vi "RGB to GRB rev.vi"(9 "ID":u8, 11 "Element":u32) -> (1 "Valid":bool, 2 "Array":bool[](array[boolean]), 3 "Reset":bool)   [LabVIEW 2016]
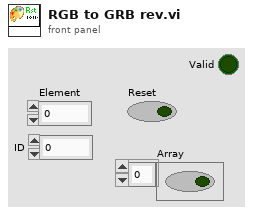
[diagram p1: front panel]
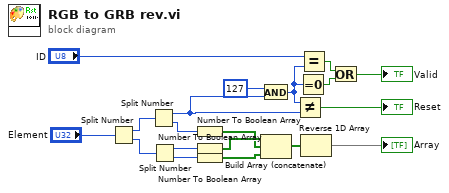
[diagram p0: block diagram]
diagram:
  n1 = Split Number(x="Element") -> (hi(x)=w12:u16, lo(x)=w13:u16)
  n2 = Split Number(x=w12) -> (hi(x)=w9:u8, lo(x)=w14:u8)
  n3 = Split Number(x=w13) -> (hi(x)=w15:u8, lo(x)=w16:u8)
  n4 = Number To Boolean Array(number=w14) -> (Boolean array=w1:bool[])
  n5 = Number To Boolean Array(number=w15) -> (Boolean array=w2:bool[])
  n6 = Number To Boolean Array(number=w16) -> (Boolean array=w17:bool[])
  n7 = And(x=u8 127, y=w9) -> (x .and. y?=w3:u8)
  n8 = Build Array (concatenate)(w2, w1, w17) -> (w18:bool[])
  n9 = Not Equal?(x=w3, y=w9) -> (x != y?=→"Reset":bool)
  n10 = Equal To 0?(x=w3) -> (x = 0?=w4:bool)
  n11 = Equal?(x="ID", y=w3) -> (x = y?=w7:bool)
  n12 = Reverse 1D Array(array=w18) -> (reversed array=→"Array":bool[])
  n13 = Or(x=w7, y=w4) -> (x .or. y?=→"Valid":bool)
